vi "例4.16 局部变量输出循环结构内的数据1.vi"() -> ()   [LabVIEW 2017]
panel:
  in  "添加的数组":i32[](array[numeric])
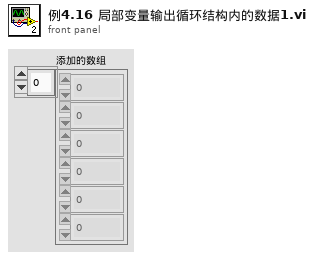
[diagram p1: front panel]
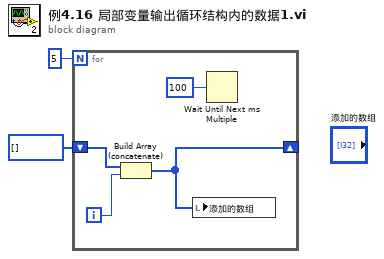
[diagram p0: block diagram]
diagram:
  n1 = for {
    N: 5 -> [_]
    shift-right: [w3] -> _
    shift-left: i32[] [] -> [w6]
    i -> [w5]
    n2 = Build Array (concatenate)(w6, w5) -> (w3:i32[])
    n3 = local write "添加的数组"(w3) -> ()
    n4 = Wait Until Next ms Multiple(millisecond multiple=u32 100 ("毫秒倍数")) -> ()  [unwired: 1 out]
  }
